vi "Generate WAMP-CRA PBKDF2-SHA-256 hash.vi"(7 "PBKDF2 serlisation method":T1, 8 "Key Length":i32=32, 9 "Iterations":i32=100, 10 "Salt":string="salt123", 11 "Secret":string="secret") -> (3 "PBKDF2 result":string="EX1Y3Q9BMM2oGLxsGqDgFeuqtPMf7Wz8Lh6PotZ62ho=")   [LabVIEW 2020, in "wamplv.lvlib"]
uses:
  wamplv.lvlib
  Private/PBKDF2 serialisation method.ctl
  Private/Authenticators/WampCraAuthenticator/WampCraAuthenticator.lvclass
panel:
  # "The WAMPs pecification does not specify how the PBKDF2 hash should be serialised\nto a string. So the wamplv library allows you to choose beteween the possible options."
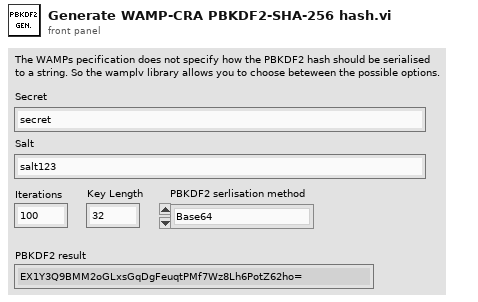
[diagram p1: front panel]
types:
  T1 = typedef "wamplv.lvlib/PBKDF2 serialisation method.ctl" = enum8{"Base64", "Hex string, lower case", "Hex string, upper case", "Direct to string cast"}
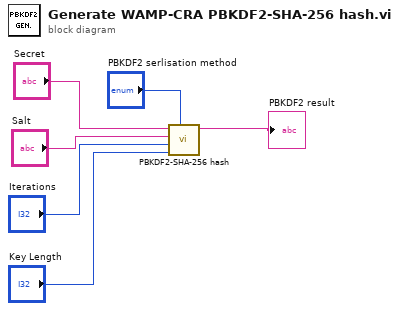
[diagram p0: block diagram]
diagram:
  n1 = call "PBKDF2-SHA-256 hash.vi"("PBKDF2 hash type"="PBKDF2 serlisation method", "Key Length"="Key Length", "Iterations"="Iterations", "Salt"="Salt", "Secret"="Secret") -> ("Hash string"=→"PBKDF2 result":string)  [unwired: 6 in]
